vi "niRFUtil WFM Parse Waveform - Span (complex wfm).vi"(3 "Span (Inf)":dbl=inf format="%^.6e", 4 "Center (0)":dbl format="%^.6e", 5 "Waveform In":T1 {"y" format="%.2f"; "dx" format="%^.2e"; "x0" format="%^.2e"}) -> (2 "Waveform Out":T1 {"y" format="%.2f"; "dx" format="%^.2e"; "x0" format="%^.2e"})   [LabVIEW 2015, in "niRFUtil.lvlib"]
doc: "(c) Copyright 2006, National Instruments, Inc. This VI may not be duplicated, sold, or distributed without written consent from National Instruments."
uses:
  niRFUtil.lvlib
  Includes/niRFUtil INC Complex Waveform.ctl
  Includes/niRFUtil INC Complex Array.ctl
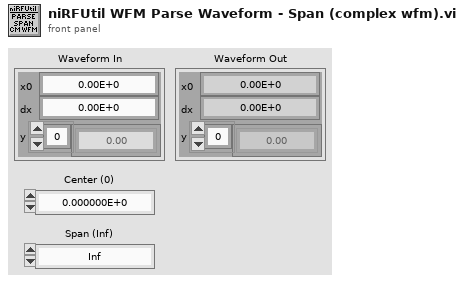
[diagram p1: front panel]
types:
  T1 = typedef "niRFUtil.lvlib/niRFUtil INC Complex Waveform.ctl" = cluster{"x0":dbl, "dx":dbl, "y":T2}
  T2 = typedef "niRFUtil.lvlib/niRFUtil INC Complex Array.ctl" = csg[]
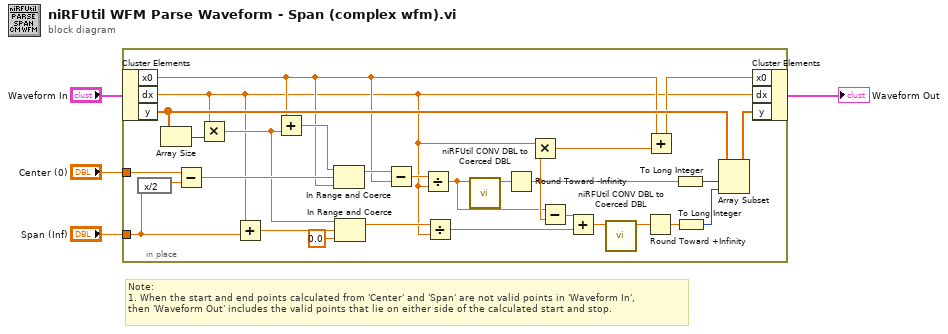
[diagram p0: block diagram]
diagram:
  # "Note:\n1. When the start and end points calculated from 'Center' and 'Span' are not valid points in 'Waveform In', \nthen 'Waveform Out' includes the valid points that lie on either side of the calculated start and stop."
  n1 = in-place {
    in-place-border: "Span (Inf)" -> [w20]
    in-place-border: "Center (0)" -> [w32]
    n2 = in-place-cluster #1("Waveform In") -> ("x0"=w15:dbl, "dx"=w13:dbl, "y"=w29:T2)
    n3 = expression code="x/2"(w20) -> (w26:dbl)
    n4 = Array Size(array=w29) -> (size(s)=w28:i32)
    n5 = Subtract(x=w32, y=w26) -> (x-y=w30:dbl)
    n6 = Multiply(x=w13, y=w28) -> (x*y=w22:dbl)
    n7 = Add(x=w13, y=w20) -> (x+y=w19:dbl)
    n8 = Add(x=w15, y=w22) -> (x+y=w27:dbl)
    n9 = In Range and Coerce(upper limit=w27, x=w30, lower limit=w15) -> (coerced(x)=w18:dbl)  [unwired: 1 out]
    n10 = In Range and Coerce(upper limit=w22, x=w19, lower limit=0.0) -> (coerced(x)=w25:dbl)  [unwired: 1 out]
    n11 = Subtract(x=w18, y=w15) -> (x-y=w14:dbl)
    n12 = Divide(x=w14, y=w13) -> (x/y=w8:dbl)
    n13 = Divide(x=w25, y=w13) -> (x/y=w24:dbl)
    n14 = call "niRFUtil CONV DBL to Coerced DBL.vi"("Numeric In (DBL)"=w8) -> ("Coerced Numeric Out (DBL)"=w7:dbl)  [unwired: 10 in]
    n15 = Round Toward -Infinity(1:w7) -> (0:w12:dbl)
    n16 = Multiply(x=w13, y=w12) -> (x*y=w16:dbl)
    n17 = Subtract(x=w8, y=w12) -> (x-y=w11:dbl)
    n18 = Add(x=w11, y=w24) -> (x+y=w6:dbl)
    n19 = call "niRFUtil CONV DBL to Coerced DBL.vi"("Numeric In (DBL)"=w6) -> ("Coerced Numeric Out (DBL)"=w5:dbl)  [unwired: 10 in]
    n20 = Round Toward +Infinity(x=w5) -> (ceil(x): smallest int >= x=w23:dbl)
    n21 = Add(x=w15, y=w16) -> (x+y=w17:dbl)
    n22 = To Long Integer(number=w12) -> (32bit integer=w10:i32)
    n23 = To Long Integer(number=w23) -> (32bit integer=w9:i32)
    n24 = Array Subset(array=w29, index=w10, length=w9) -> (w31:T2)
    n25 = in-place-cluster #1("x0"=w17, "dx"=w13, "y"=w31) -> (→"Waveform Out":T1)
  }
